vi "Task_issue.vi"() -> ()   [LabVIEW 2023]
uses:
  <vilib>/DAQmx/read.llb/DAQmx Read (Analog Wfm 1Chan NSamp).vi
  <vilib>/DAQmx/create/channels.llb/DAQmx Create Channel (AI-Temperature-Thermocouple).vi
  <vilib>/DAQmx/configure/timing.llb/DAQmx Timing (Sample Clock).vi
  <vilib>/DAQmx/miscellaneous.llb/DAQmx Fill In Error Info.vi
  <vilib>/Waveform/WDTOps.llb/WDT Number of Waveform Samples DBL.vi
  <resource>/objmgr/daqmx.rc
panel:
  out "sum samples 2":i32
  out "sum samples":i32
  out "Waveform Chart 2":waveform(dbl)(graph)
  out "Waveform Chart":waveform(dbl)(graph)
  out "error in (no error)":errorcluster
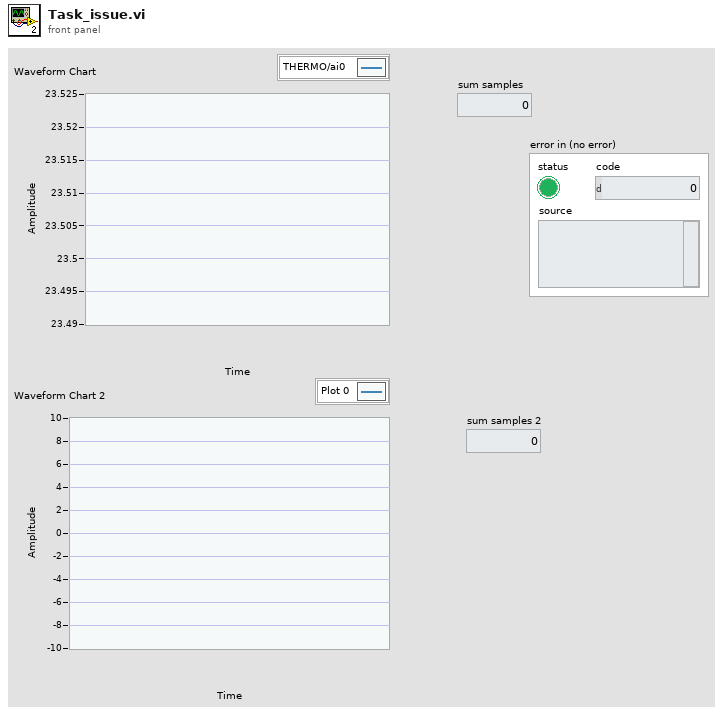
[diagram p1: front panel]
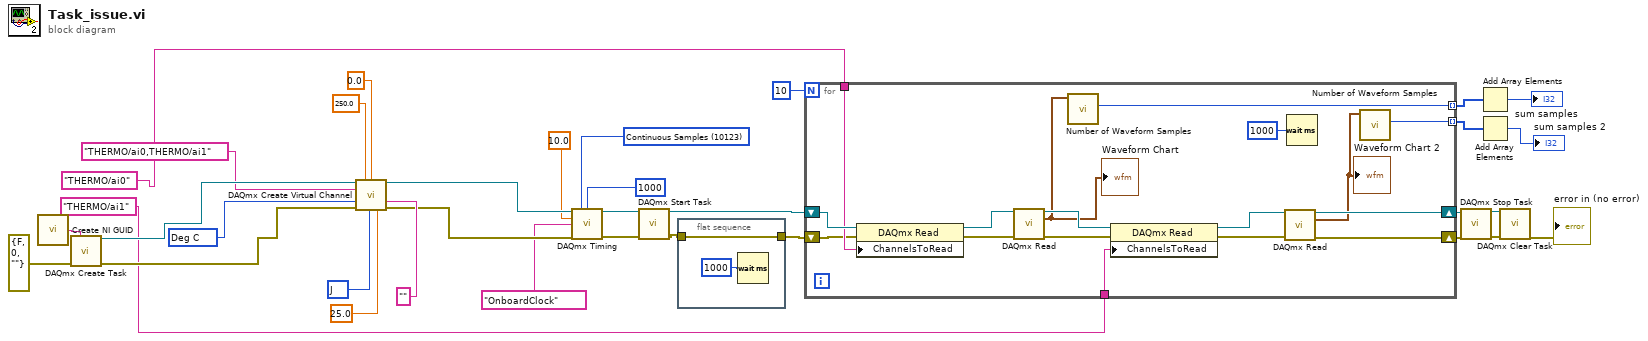
[diagram p0: block diagram]
diagram:
  w8 = 10123 items=["Finite Samples"=10178, "Continuous Samples"=10123, "Hardware Timed Single Point"=12522] ("sample mode")
  w28 = 10072 items=["J"=10072, "K"=10073, "N"=10077, "R"=10082, "S"=10085, "T"=10086, "B"=10047, "E"=10055] ("thermocouple type")
  w32 = 10143 items=["Deg C"=10143, "Deg F"=10144, "Kelvins"=10325, "Deg R"=10145, "From Custom Scale"=10065] ("units")
  n1 = call <vilib>:"Create NI GUID.vi"() -> ("NI GUID"=w22:string)
  n2 = call <vilib>:"DAQmx Create Task.vi"("new task name"=w22, "error in"=errorcluster {"status"=FALSE, "code"=0, "source"=""} ("error in (no error)")) -> ("task out"=w21:refnum<k21>, "error out"=w23:errorcluster)  [unwired: 12 in]
  n3 = call-poly <vilib>:"DAQmx Create Virtual Channel.vi"("task in"=w21, "maximum value"=250.0, "minimum value"=0.0 ("maximum value"), "physical channels"="THERMO/ai0,THERMO/ai1", "units"=w32, "cjc channel"="", "error in"=w23, "thermocouple type"=w28, "cjc value"=25.0 ("maximum value")) -> ("task out"=w25:refnum<k21>, "error out"=w27:errorcluster)  [unwired: 5 in]
  n4 = call-poly <vilib>:"DAQmx Timing.vi"("task/channels in"=w25, "sample mode"=w8, "samples per channel"=1000, "rate"=10.0, "source"=tag "OnboardClock", "error in"=w27) -> ("task out"=w20:refnum<k21>, "error out"=w26:errorcluster)  [unwired: 8 in]
  n5 = call <vilib>:"DAQmx Start Task.vi"("task/channels in"=w20, "error in"=w26) -> ("task out"=w16:refnum<k21>, "error out"=w11:errorcluster)  [unwired: 12 in]
  n6 = flat-sequence {
    tunnel: [w36] -> w12
    tunnel: w11 -> [w36]
    frame #0 {
      n7 = Wait (ms)(milliseconds to wait=u32 1000) -> ()  [unwired: 1 out]
    }
  }
  n8 = for {
    N: 10 -> [_]
    tunnel: "THERMO/ai0" -> [w50]
    tunnel: "THERMO/ai1" -> [w42]
    shift-right: [w48] -> w14
    shift-left: w16 -> [w52]
    shift-right: [w47] -> w13
    shift-left: w12 -> [w46]
    tunnel: [w39] -> w5 mode=indexing
    tunnel: [w37] -> w3 mode=indexing
    n9 = property class="DAQmx Read"(reference=w52, error in=w46, "ChannelsToRead"=w50) -> (reference out=w51:refnum<k21>, error out=w53:errorcluster)
    n10 = call-poly <vilib>:"DAQmx Read.vi"("task/channels in"=w51, "error in"=w53) -> ("task out"=w49:refnum<k21>, "data"=w40:waveform(dbl), "error out"=w44:errorcluster)  [unwired: 11 in]
    "Waveform Chart" <- w40
    n11 = call-poly <vilib>:"Number of Waveform Samples.vi"("waveform in"=w40) -> ("number of samples"=w39:i32)  [unwired: 8 in, 2 out]
    n12 = property class="DAQmx Read"(reference=w49, error in=w44, "ChannelsToRead"=w42) -> (reference out=w45:refnum<k21>, error out=w43:errorcluster)
    n13 = call-poly <vilib>:"DAQmx Read.vi"("task/channels in"=w45, "error in"=w43) -> ("task out"=w48:refnum<k21>, "data"=w38:waveform(dbl), "error out"=w47:errorcluster)  [unwired: 11 in]
    "Waveform Chart 2" <- w38
    n14 = Wait (ms)(milliseconds to wait=u32 1000) -> ()  [unwired: 1 out]
    n15 = call-poly <vilib>:"Number of Waveform Samples.vi"("waveform in"=w38) -> ("number of samples"=w37:i32)  [unwired: 8 in, 2 out]
  }
  n16 = call <vilib>:"DAQmx Stop Task.vi"("task/channels in"=w14, "error in"=w13) -> ("task out"=w17:refnum<k21>, "error out"=w19:errorcluster)  [unwired: 12 in]
  n17 = Add Array Elements(numeric array=w5) -> (sum=→"sum samples":i32)
  n18 = Add Array Elements(numeric array=w3) -> (sum=→"sum samples 2":i32)
  n19 = call <vilib>:"DAQmx Clear Task.vi"("task in"=w17, "error in"=w19) -> ("error out"=→"error in (no error)":errorcluster)  [unwired: 13 in]
